vi "viewerDisplay.vi"(8 "error in (no error)":errorcluster, 11 "ImageStreamViewer in":refnum<class "ImageStreamViewer.lvclass">) -> (0 "error out":errorcluster, 3 "ImageStreamViewer out":refnum<class "ImageStreamViewer.lvclass">)   [LabVIEW 2011, in "Views.lvlib" / "Camera.lvlib" / "ImageStreamViewer.lvclass"]
uses:
  ImageStreamViewer.lvclass
  ImageStreamViewer.lvclass/ImageStreamViewer.ctl
panel:
  in  "Slide":dbl(slide)=1604.0 scale=0.0..4236.0
  in  "stop":bool
  out "y profile":cluster{"Pixels Line":sgl[], i32[]}(graph)
  out "X Profile":cluster{"x0":sgl, "dx":sgl, "Pixels Line":sgl[]}(graph)
  in  "Scrollbar":i32(c297)
  out "Path":path
  out "Image":T1(plugin-control)
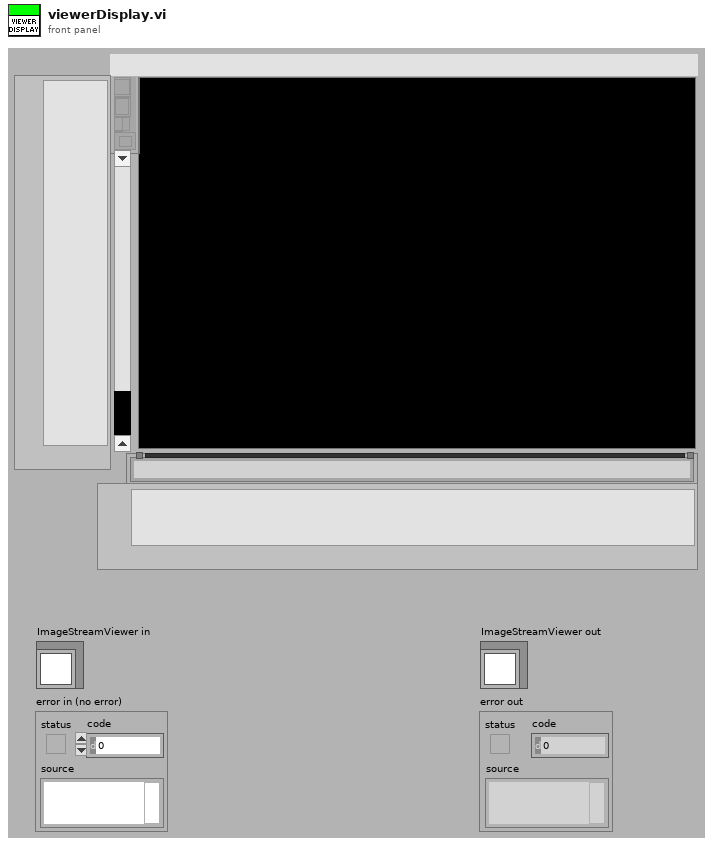
[diagram p1: front panel]
types:
  T1 = typedef "IMAQ Image.ctl" = refnum<image>
  T2 = typedef "LVPoint32TypeDef.ctl" = cluster{"Horizontal":i32, "Vertical":i32}
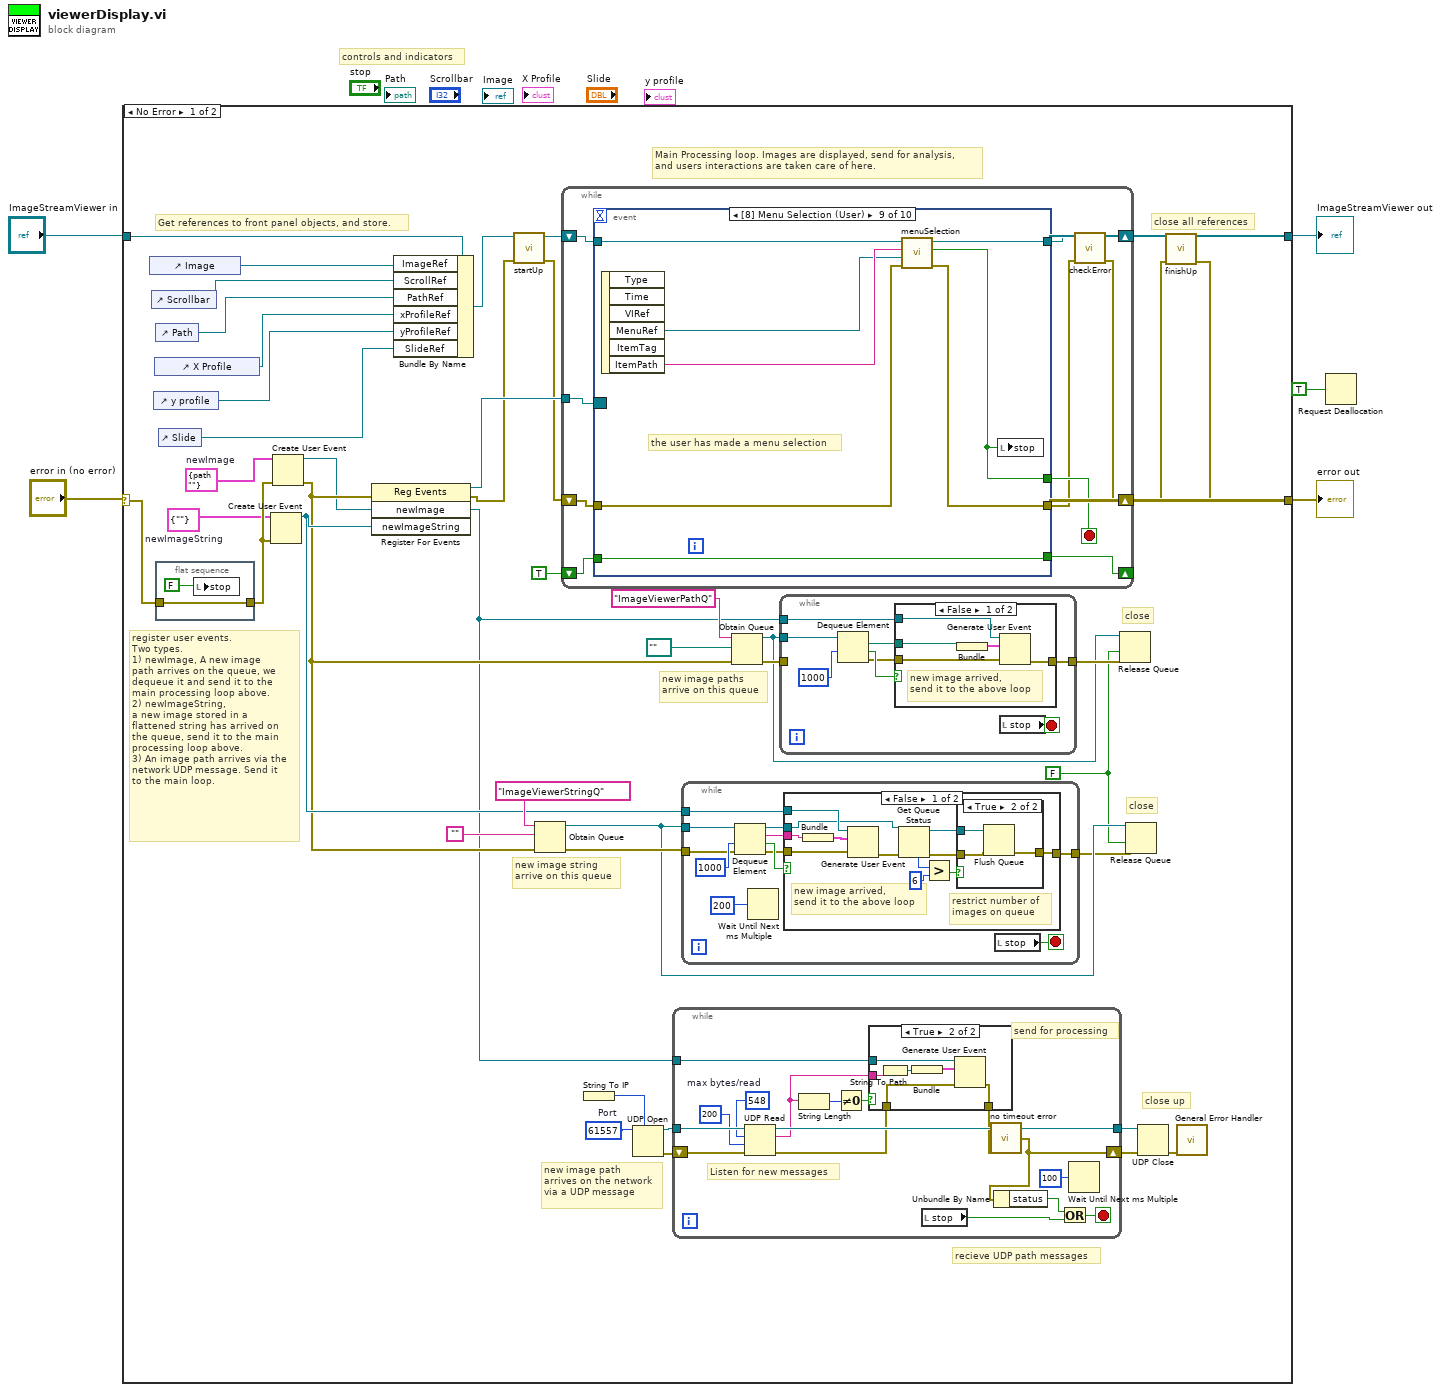
[diagram p0: block diagram]
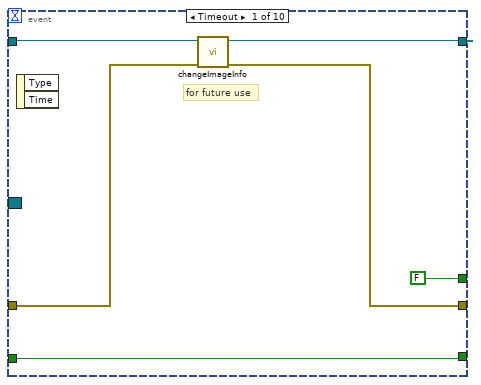
[diagram p6: hidden frame]
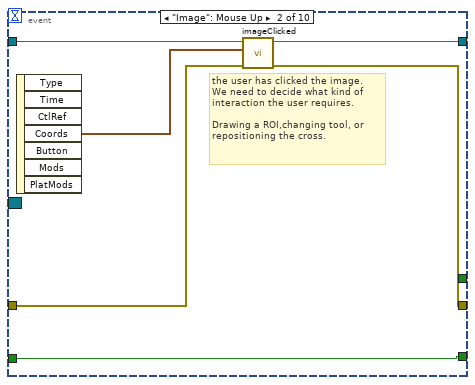
[diagram p7: hidden frame]
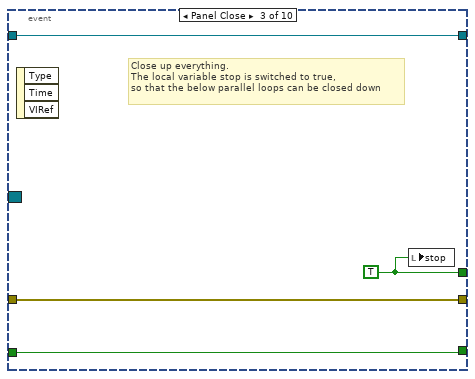
[diagram p8: hidden frame]
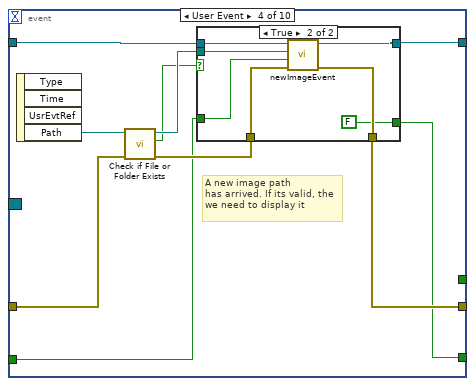
[diagram p9: hidden frame]
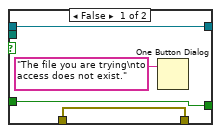
[diagram p10: hidden frame]
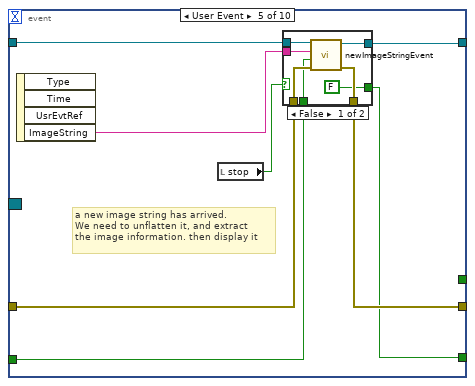
[diagram p11: hidden frame]
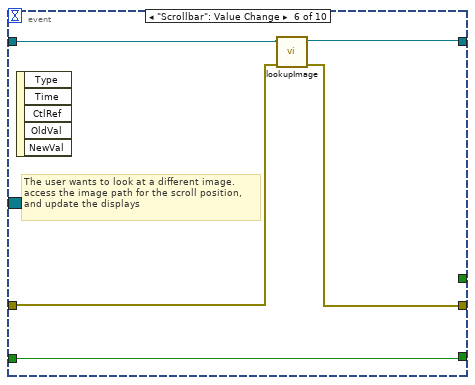
[diagram p13: hidden frame]
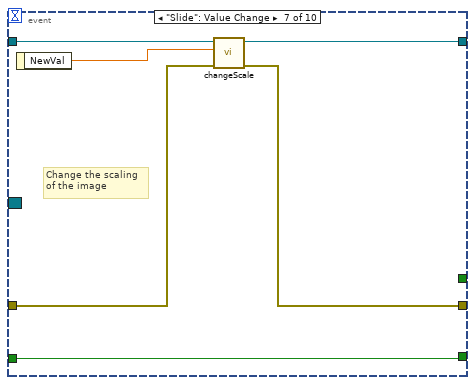
[diagram p14: hidden frame]
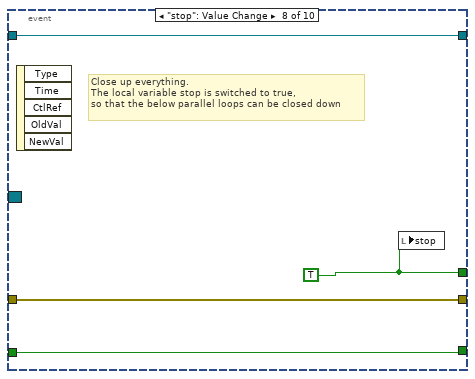
[diagram p15: hidden frame]
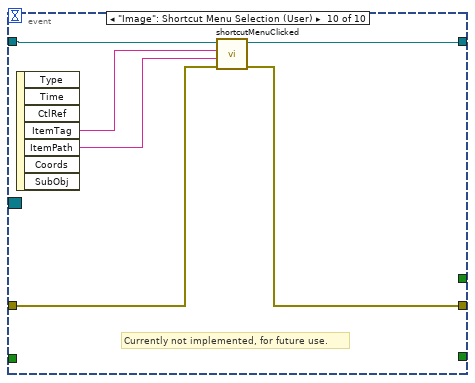
[diagram p16: hidden frame]
diagram:
  # "controls and indicators"
  n1 = case shown="No Error" "error in (no error)" {
    selector: "error in (no error)" -> [w42 w210]
    tunnel: [w27 w210] -> w4
    tunnel: [w29 w209] -> w2
    tunnel: "ImageStreamViewer in" -> [w41 w209]
    frame No Error {
      w10 = u16 61557  # Port
      w23 = FALSE
      w32 = cluster{"ImageString":string} {"ImageString"=""}  # newImageString
      w46 = cluster{"Path":path} {"Path"=path ""}  # newImage
      # "Main Processing loop. Images are displayed, send for analysis,\nand users interactions are taken care of here."
      # "close"
      # "close"
      # "close up"
      # "new image path\narrives on the network\nvia a UDP message"
      # "close all references"
      # "register user events.\nTwo types.\n1) newImage, A new image\npath arrives on the queue, we\ndequeue it and send it to the\nmain processing loop above.\n2) newImageString,\na new image stored in a\nflattened string has arrived on\nthe queue, send it to the main\nprocessing loop above.\n3) An image path arrives via the\nnetwork UDP message. Send it \nto the main loop."
      # "Get references to front panel objects, and store."
      # "recieve UDP path messages"
      # "new image string\narrive on this queue"
      # "new image paths\narrive on this queue"
      n2 = control-ref of="Image"() -> (w17:refnum<vi>)
      n3 = control-ref of="Scrollbar"() -> (w40:refnum<vi>)
      n4 = control-ref of="y profile"() -> (w37:refnum<vi>)
      n5 = control-ref of="X Profile"() -> (w38:refnum<vi>)
      n6 = control-ref of="Path"() -> (w39:refnum<vi>)
      n7 = flat-sequence {
        tunnel: w42 -> [w99]
        tunnel: [w99] -> w33
        frame #0 {
          n8 = local write "stop"(FALSE) -> ()
        }
      }
      n9 = control-ref of="Slide"() -> (w7:refnum<vi>)
      n10 = Create User Event(user event datatype=w32, error in=w33) -> (user event=w31:refnum<user-event>)  [unwired: 1 out]
      n11 = Create User Event(user event datatype=w46, error in=w33) -> (user event=w9:refnum<user-event>, error out=w18:errorcluster)
      n12 = register-events(error in=w18, w9, w31) -> (reference out=w47:refnum<event-registration>, error out=w20:errorcluster)  [unwired: 1 in]
      n13 = Bundle By Name(cluster=w41, "ImageRef"=w17, "ScrollRef"=w40, "PathRef"=w39, "xProfileRef"=w38, "yProfileRef"=w37, "SlideRef"=w7) -> (w22:refnum<class "ImageStreamViewer.lvclass">)
      n14 = call "startUp.vi"("error in (no error)"=w20, "ImageStreamViewer in"=w22) -> ("error out"=w19:errorcluster, "ImageStreamViewer out"=w21:refnum<class "ImageStreamViewer.lvclass">)  [unwired: 8 in]
      n15 = Obtain Queue(name (unnamed)="ImageViewerStringQ", element data type="", error in (no error)=w18) -> (queue out=w26:refnum<queue>, error out=w34:errorcluster)  [unwired: 2 in, 1 out]
      n16 = while {
        shift-right: [w119] -> w30
        shift-left: w21 -> [w124]
        shift-right: [w117] -> w28
        shift-left: w19 -> [w123]
        tunnel: w47 -> [w121]
        shift-right: [w115] -> _
        shift-left: TRUE -> [w116]
        stop <- w122 stop-if-true
        n17 = event shown="[8] Menu Selection (User)" {
          selector: w121 -> [_ _ _ _ _ _ _ _ _ _]
          dyn-events: _ -> [_ _ _ _ _ _ _ _ _ _]
          timeout: _ -> [_ _ _ _ _ _ _ _ _ _]
          tunnel: w124 -> [w129 w136 w140 w150 w169 w184 w190 w192 w202 w208]
          tunnel: w123 -> [w127 w135 w138 w144 w166 w182 w188 w194 w200 w204]
          tunnel: [w128 w133 w140 w149 w168 w183 w189 w192 w201 w207] -> w120
          tunnel: [w125 w134 w138 w148 w165 w181 w187 w194 w199 w203] -> w118
          tunnel: [FALSE _ w139 _ _ _ _ w193 w197 _] -> w122
          tunnel: w116 -> [w126 w131 w137 w141 w163 w180 w185 w191 w195 _]
          tunnel: [w126 w131 w137 w142 w162 w180 w185 w191 w195 _] -> w115
          event Timeout {
            # "for future use"
            n18 = event-data() -> ()  [unwired: 1 in, 2 out]
            n19 = call "changeImageInfo.vi"("error in (no error)"=w127, "ImageStreamViewer in"=w129) -> ("error out"=w125:errorcluster, "ImageStreamViewer out"=w128:refnum<class "ImageStreamViewer.lvclass">)  [unwired: 8 in]
          }
          event "Image": Mouse Up {
            # "the user has clicked the image.\nWe need to decide what kind of \ninteraction the user requires. \n\nDrawing a ROI,changing tool, or \nrepositioning the cross."
            n20 = event-data() -> ("Coords"=w132:T2)  [unwired: 1 in, 6 out]
            n21 = call "imageClicked.vi"("error in (no error)"=w135, "Point"=w132, "ImageStreamViewer in"=w136) -> ("error out"=w134:errorcluster, "ImageStreamViewer out"=w133:refnum<class "ImageStreamViewer.lvclass">)  [unwired: 7 in]
          }
          event Panel Close {
            w139 = TRUE
            # "Close up everything.\nThe local variable stop is switched to true,\nso that the below parallel loops can be closed down"
            n22 = event-data() -> ()  [unwired: 1 in, 3 out]
            n23 = local write "stop"(w139) -> ()
          }
          event User Event {
            # "A new image path\nhas arrived. If its valid, the\nwe need to display it"
            n24 = event-data() -> ("Path"=w147:path)  [unwired: 1 in, 3 out]
            n25 = call <vilib>:"Check if File or Folder Exists.vi"("error in (no error)"=w144, "path"=w147) -> ("error out"=w143:errorcluster, "file or folder exists?"=w145:bool, "dup path"=w146:path)  [unwired: 7 in]
            n26 = case shown="True" w145 {
              tunnel: w150 -> [w154 w161]
              tunnel: [w154 w160] -> w149
              tunnel: [w153 w159] -> w148
              tunnel: w143 -> [w153 w158]
              tunnel: w146 -> [_ w157]
              tunnel: [w151 FALSE] -> w142
              tunnel: w141 -> [w151 w155]
              frame False {
                n27 = One Button Dialog(message="The file you are trying\nto access does not exist.") -> ()  [unwired: 1 in, 1 out]
              }
              frame True {
                n28 = call "newImageEvent.vi"("error in (no error)"=w158, "firstImage?"=w155, "Path"=w157, "ImageStreamViewer in"=w161) -> ("error out"=w159:errorcluster, "ImageStreamViewer out"=w160:refnum<class "ImageStreamViewer.lvclass">)  [unwired: 6 in]
              }
            }
          }
          event User Event {
            # "a new image string has arrived. \nWe need to unflatten it, and extract \nthe image information. then display it"
            n29 = event-data() -> ("ImageString"=w167:string)  [unwired: 1 in, 3 out]
            n30 = local read "stop"() -> (w164:bool)
            n31 = case shown="False" w164 {
              tunnel: w169 -> [w176 w179]
              tunnel: [w175 w179] -> w168
              tunnel: w167 -> [w174 _]
              tunnel: w166 -> [w173 w178]
              tunnel: [w172 w178] -> w165
              tunnel: w163 -> [w170 w177]
              tunnel: [FALSE w177] -> w162
              frame False {
                n32 = call "newImageStringEvent.vi"("error in (no error)"=w173, "firstImage?"=w170, "ImageString"=w174, "ImageStreamViewer in"=w176) -> ("error out"=w172:errorcluster, "ImageStreamViewer out"=w175:refnum<class "ImageStreamViewer.lvclass">)  [unwired: 6 in]
              }
              frame True {
              }
            }
          }
          event "Scrollbar": Value Change {
            # "The user wants to look at a different image.\naccess the image path for the scroll position,\nand update the displays"
            n33 = event-data() -> ()  [unwired: 1 in, 5 out]
            n34 = call "lookupImage.vi"("error in (no error)"=w182, "ImageStreamViewer in"=w184) -> ("error out"=w181:errorcluster, "ImageStreamViewer out"=w183:refnum<class "ImageStreamViewer.lvclass">)  [unwired: 8 in]
          }
          event "Slide": Value Change {
            # "Change the scaling\nof the image"
            n35 = event-data() -> ("NewVal"=w186:dbl)  [unwired: 1 in]
            n36 = call "changeScale.vi"("error in (no error)"=w188, "newValue"=w186, "ImageStreamViewer in"=w190) -> ("error out"=w187:errorcluster, "ImageStreamViewer out"=w189:refnum<class "ImageStreamViewer.lvclass">)  [unwired: 7 in]
          }
          event "stop": Value Change {
            w193 = TRUE
            # "Close up everything.\nThe local variable stop is switched to true,\nso that the below parallel loops can be closed down"
            n37 = event-data() -> ()  [unwired: 1 in, 5 out]
            n38 = local write "stop"(w193) -> ()
          }
          event Menu Selection (User) {
            # "the user has made a menu selection"
            n39 = event-data() -> ("MenuRef"=w196:refnum<k9>, "ItemPath"=w198:string)  [unwired: 1 in, 4 out]
            n40 = call "menuSelection.vi"("error in (no error)"=w200, "MenuRef"=w196, "itemPath"=w198, "ImageStreamViewer in"=w202) -> ("error out"=w199:errorcluster, "close"=w197:bool, "ImageStreamViewer out"=w201:refnum<class "ImageStreamViewer.lvclass">)  [unwired: 5 in]
            n41 = local write "stop"(w197) -> ()
          }
          event "Image": Shortcut Menu Selection (User) {
            # "Currently not implemented, for future use."
            n42 = event-data() -> ("ItemTag"=w206:string, "ItemPath"=w205:string)  [unwired: 1 in, 5 out]
            n43 = call "shortcutMenuClicked.vi"("error in (no error)"=w204, "path"=w205, "tag"=w206, "ImageStreamViewer in"=w208) -> ("error out"=w203:errorcluster, "ImageStreamViewer out"=w207:refnum<class "ImageStreamViewer.lvclass">)  [unwired: 6 in]
          }
        }
        n44 = call "checkError.vi"("error in (no error)"=w118, "ImageStreamViewer in"=w120) -> ("error out"=w117:errorcluster, "ImageStreamViewer out"=w119:refnum<class "ImageStreamViewer.lvclass">)  [unwired: 8 in]
      }
      n45 = String To IP() -> (0:w8:u32)  [unwired: 1 in]
      n46 = UDP Open(7:w8, 11:w10) -> (port=w12:refnum<k16>, 0:w11:errorcluster)  [unwired: 3 in, 1 out]
      n47 = while {
        tunnel: [w61] -> w13
        tunnel: w12 -> [w62]
        shift-left: w11 -> [w63]
        shift-right: [w57] -> w14
        tunnel: w9 -> [w49]
        stop <- w59 stop-if-true
        w56 = 548  # max bytes/read
        # "send for processing"
        # "Listen for new messages"
        n48 = UDP Read(connection ID=w62, max size (548)=w56, timeout ms (25000)=200, 8:w63) -> (data out=w54:string, error out=w51:errorcluster, 3:w61:refnum<k16>)  [unwired: 2 out]
        n49 = String Length(string=w54) -> (length=w53:i32)
        n50 = Not Equal To 0?(x=w53) -> (x != 0?=w52:bool)
        n51 = case shown="True" w52 {
          tunnel: w54 -> [_ w67]
          tunnel: w51 -> [w64 w69]
          tunnel: [w64 w68] -> w50
          tunnel: w49 -> [_ w65]
          frame False {
          }
          frame True {
            n52 = String To Path(string=w67) -> (path=w66:path)
            n53 = Bundle(w66) -> (w70:cluster{path})  [unwired: 1 in]
            n54 = Generate User Event(user event=w65, event data cluster=w70, error in=w69) -> (error out=w68:errorcluster)  [unwired: 1 out]
          }
        }
        n55 = local read "stop"() -> (w48:bool)
        n56 = call "no timeout error.vi"("error in (no error)"=w50) -> ("error out"=w57:errorcluster)
        n57 = Unbundle By Name(w57) -> ("status"=w58:bool)
        n58 = Or(x=w58, y=w48) -> (x .or. y?=w59:bool)
        n59 = Wait Until Next ms Multiple(millisecond multiple=u32 100) -> ()  [unwired: 1 out]
      }
      n60 = while {
        tunnel: w31 -> [w78]
        tunnel: w34 -> [w75]
        tunnel: w26 -> [w74]
        tunnel: [w72] -> w16
        stop <- w77 stop-if-true
        n61 = Dequeue Element(queue=w74, timeout in ms (-1)=1000, error in (no error)=w75) -> (queue out=w73:refnum<queue>, element=w76:string, timed out?=w80:bool, error out=w79:errorcluster)
        n62 = Wait Until Next ms Multiple(millisecond multiple=200) -> ()  [unwired: 1 out]
        n63 = case shown="False" w80 {
          tunnel: w79 -> [w93 w98]
          tunnel: w78 -> [w92 _]
          tunnel: [w82 w98] -> w72
          tunnel: w76 -> [w90 _]
          tunnel: w73 -> [w88 _]
          frame False {
            # "restrict number of \nimages on queue"
            # "new image arrived, \nsend it to the above loop"
            n64 = Bundle(w90) -> (w91:cluster{string})  [unwired: 1 in]
            n65 = Generate User Event(user event=w92, event data cluster=w91, error in=w93) -> (error out=w89:errorcluster)  [unwired: 1 out]
            n66 = Get Queue Status(queue=w88, error in (no error)=w89) -> (queue out=w84:refnum<queue>, error out=w83:errorcluster, # elements in queue=w87:i32)  [unwired: 1 in, 5 out]
            n67 = Greater?(x=w87, y=6) -> (0:w85:bool)
            n68 = case shown="True" w85 {
              tunnel: w84 -> [_ w97]
              tunnel: w83 -> [w94 w96]
              tunnel: [w94 w95] -> w82
              frame False {
              }
              frame True {
                n69 = Flush Queue(queue=w97, error in (no error)=w96) -> (error out=w95:errorcluster)  [unwired: 2 out]
              }
            }
          }
          frame True {
            # "timeout"
          }
        }
        n70 = local read "stop"() -> (w77:bool)
      }
      n71 = Obtain Queue(name (unnamed)="ImageViewerPathQ", element data type=path "", error in (no error)=w18) -> (queue out=w24:refnum<queue>, error out=w43:errorcluster)  [unwired: 2 in, 1 out]
      n72 = while {
        tunnel: w9 -> [w103]
        tunnel: w24 -> [w108]
        tunnel: w43 -> [_]
        tunnel: [w102] -> w25
        stop <- w101 stop-if-true
        n73 = Dequeue Element(queue=w108, timeout in ms (-1)=1000) -> (element=w105:path, timed out?=w106:bool, error out=w104:errorcluster)  [unwired: 1 in, 1 out]
        n74 = case shown="False" w106 {
          tunnel: w105 -> [w110 _]
          tunnel: w104 -> [w113 w114]
          tunnel: w103 -> [w112 _]
          tunnel: [w109 w114] -> w102
          frame False {
            # "new image arrived, \nsend it to the above loop"
            n75 = Bundle(w110) -> (w111:cluster{path})  [unwired: 1 in]
            n76 = Generate User Event(user event=w112, event data cluster=w111, error in=w113) -> (error out=w109:errorcluster)  [unwired: 1 out]
          }
          frame True {
            # "timeout"
          }
        }
        n77 = local read "stop"() -> (w101:bool)
      }
      n78 = Release Queue(queue=w24, force destroy? (F)=w23, error in (no error)=w25) -> ()  [unwired: 3 out]
      n79 = Release Queue(queue=w26, force destroy? (F)=w23, error in (no error)=w16) -> ()  [unwired: 3 out]
      n80 = UDP Close(connection ID=w13, 8:w14) -> (error out=w15:errorcluster)  [unwired: 1 out]
      n81 = call "finishUp.vi"("error in (no error)"=w28, "ImageStreamViewer in"=w30) -> ("error out"=w27:errorcluster, "ImageStreamViewer out"=w29:refnum<class "ImageStreamViewer.lvclass">)  [unwired: 8 in]
      n82 = call <vilib>:"General Error Handler.vi"("error in (no error)"=w15) -> ()  [unwired: 10 in, 5 out]
    }
    frame Error {
    }
  }
  "error out" <- w4
  "ImageStreamViewer out" <- w2
  n83 = Request Deallocation(TRUE ("flag")) -> ()
